vi "Uninitialize Analysis Workspace.vi"(8 "error in (no error)":errorcluster) -> (0 "error out":errorcluster)   [LabVIEW 2010, in "NI_AALPro.lvlib"]
doc: "Releases all resources used by the analysis workspace. To prevent race conditions, priority inversions, and other undefined behavior, you must use the Uninitialize Analysis Workspace VI according to a strict set of guidelines."
uses:
  NI_AALPro.lvlib
  lvanlys.dll
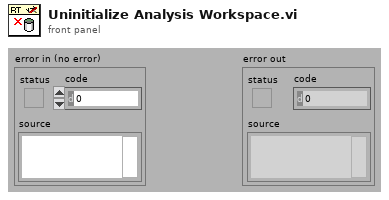
[diagram p1: front panel]
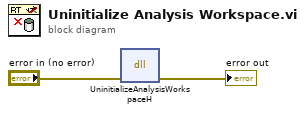
[diagram p0: block diagram]
diagram:
  n1 = dll-call lib="C:/Program Files/National Instruments/LabVIEW 2010/resource/lvanlys.*" fn="UninitializeAnalysisWorkspaceH"("_errorCluster"="error in (no error)") -> ("_errorCluster"=→"error out":errorcluster)  [unwired: 4 in, 2 out]
